vi "Pack Return Msg.vi"(11 "Dialog Return Msg in":refnum<class "Dialog Return Msg.lvclass">) -> (3 "Dialog Return Msg out":refnum<class "Dialog Return Msg.lvclass">)   [LabVIEW 2019, in "IDialogBox.lvlib" / "Dialog Return Msg.lvclass"]
uses:
  <vilib>/gpm_packages/@cs/mva-dialogbox/source/IDialogBox/IDialogBox Messages/Dialog Return Msg/Dialog Return Msg.lvclass
  C:/Program Files/National Instruments/LabVIEW 2019/vi.lib/gpm_packages/@cs/actor-framework-messages/Source/RoundTripMessage/RoundTripMessage.lvclass
  <vilib>/ActorFramework/Message Enqueuer/Message Enqueuer.lvclass
  <vilib>/ActorFramework/Message Enqueuer/Message Priority.ctl
  <vilib>/gpm_packages/@cs/actor-framework-messages/Source/RoundTripMessage/RoundTripMessage.lvclass/RoundTripMessage.ctl
  <vilib>/gpm_packages/@cs/actor-framework-messages/Source/RoundTripMessage/RoundTripMessage.lvclass
panel:
  in  "Return Priority (Normal)":T1=enum."Normal"
  in  "Return Address":refnum<class "Message Enqueuer.lvclass">
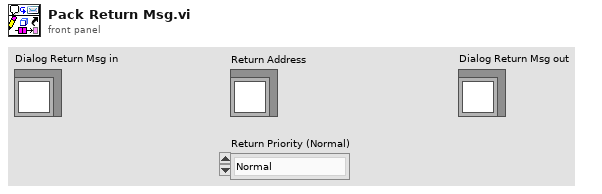
[diagram p1: front panel]
types:
  T1 = typedef "Actor Framework.lvlib/Message Enqueuer.lvclass/Message Priority.ctl" = enum16{"Low", "Normal", "High"}
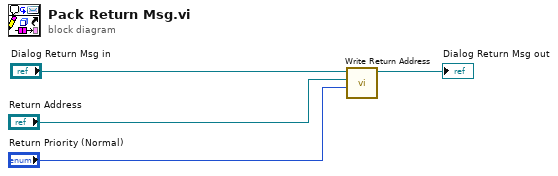
[diagram p0: block diagram]
diagram:
  n1 = call <vilib>:"Write Return Address.vi"("Return Priority (Normal)"="Return Priority (Normal)", "Return Enqueuer"="Return Address", "RoundTripMessage In"="Dialog Return Msg in") -> ("RoundTripMessage Out"=→"Dialog Return Msg out":refnum<class "Dialog Return Msg.lvclass">)  [unwired: 8 in]
